vi "Sub.vi"(10 "B":dbl, 11 "A":dbl) -> (3 "C":dbl)   [LabVIEW 2018]
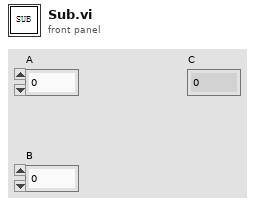
[diagram p1: front panel]
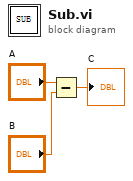
[diagram p0: block diagram]
diagram:
  n1 = Subtract(x="A", y="B") -> (x-y=→"C":dbl)
